vi "ScanPi.vi"() -> ()   [LabVIEW 2019]
uses:
  <vilib>/Platform/TimedLoop/XDataNode/timing_clust.ctl
  <vilib>/Platform/TimedLoop/XDataNode/nitl_modes.ctl
  <vilib>/Platform/TimedLoop/XDataNode/wakeup.ctl
  <vilib>/Analysis/6fits.llb/Curve Fitting Criteria.ctl
  <vilib>/DAQmx/write.llb/DAQmx Write (Analog Wfm 1Chan NSamp).vi
  <vilib>/DAQmx/read.llb/DAQmx Read (Analog Wfm 1Chan NSamp).vi
  <vilib>/Analysis/baseanly.llb/Mean (DBL).vi
  <vilib>/DAQmx/create/channels.llb/DAQmx Create Channel (AO-Voltage-Basic).vi
  <vilib>/DAQmx/configure/timing.llb/DAQmx Timing (Sample Clock).vi
  <vilib>/DAQmx/miscellaneous.llb/DAQmx Fill In Error Info.vi
  <vilib>/DAQmx/create/channels.llb/DAQmx Create Channel (AI-Voltage-Basic).vi
  <vilib>/measure/mascope.llb/Amplitude and Levels 1 chan.vi
  <vilib>/Utility/file.llb/Write Delimited Spreadsheet (DBL).vi
  <vilib>/gmath/NumericalOptimization/Nonlinear Curve Fit LM formula string.vi
  <vilib>/platform/TimedLoop/XDataNode/XDataNode.xnode
  <vilib>/Analysis/NI_AALBase.lvlib
  <vilib>/Platform/TimedLoop/XDataNode/XDNodeRunTimeDep.lvlib
  <vilib>/gmath/NI_Gmath.lvlib
  <vilib>/measure/NI_MABase.lvlib
  <vilib>/measure/NI_MAPro.lvlib
  <vilib>/Analysis/NI_AALPro.lvlib
panel:
  in  "VoltGuess":dbl format="%#_13g"
  in  "file path (dialog if empty)":path=path "C:/Users/Weak/Desktop/May_2018/newAlignment/gpHA_-1185_-1132_31deg.csv"
  in  "stop 2":bool
  in  "Phase":dbl=31.0
  out "In Range?":bool=TRUE
  out "element":dbl=0.7624557364514131
  in  "Ki":dbl=0.15
  in  "Kp":dbl=0.04
  out "m":dbl=-3.5466103770531032
  out "offset":dbl=-1.2655842803924016
  out "Waveform Chart":dynamicdata(graph)=[{"t0"=timestamp(3609575742.2676673 s since 1904-01-01), "dt"=1.0, "Y"=[-6.117337894946104]}, {"t0"=timestamp(3609575742.255667 s since 1904-01-01), "dt"=1.0, "Y"=[-6.086605623645964]}, {"t0"=timestamp(3609575742.2676673 s since 1904-01-01), "dt"=1.0, "Y"=[-1.7123814874696823]}, {"t0"=timestamp(3609575742.2676673 s since 1904-01-01), "dt"=1.0, "Y"=[-0.030732271300140113]}]
  in  "stop":bool
  out "Scanning":waveform(dbl)[](graph)=[{"t0"=timestamp(0 s since 1904-01-01), "dt"=0.000333325, "Y"=array[3000 elements]}, {"t0"=timestamp(0 s since 1904-01-01), "dt"=0.0003333333333333333, "Y"=array[3000 elements]}, {"t0"=timestamp(0 s since 1904-01-01), "dt"=0.000333325, "Y"=array[3000 elements], "attributes"=variant("NI_ChannelName"=variant(string "Filtered (Filtered)"), "NI_OriginalChannelName"=variant(string "Filtered"))}]
  in  "stop Lock":bool
  out "Locking":cluster{"Y":dbl[], "best nonlinear fit":dbl[]}[](graph)=[{"Y"=[-1.2487077639208923], "best nonlinear fit"=[-6.086605623645964]}, {"Y"=array[214 elements], "best nonlinear fit"=array[214 elements]}, {"Y"=array[214 elements], "best nonlinear fit"=array[214 elements]}]
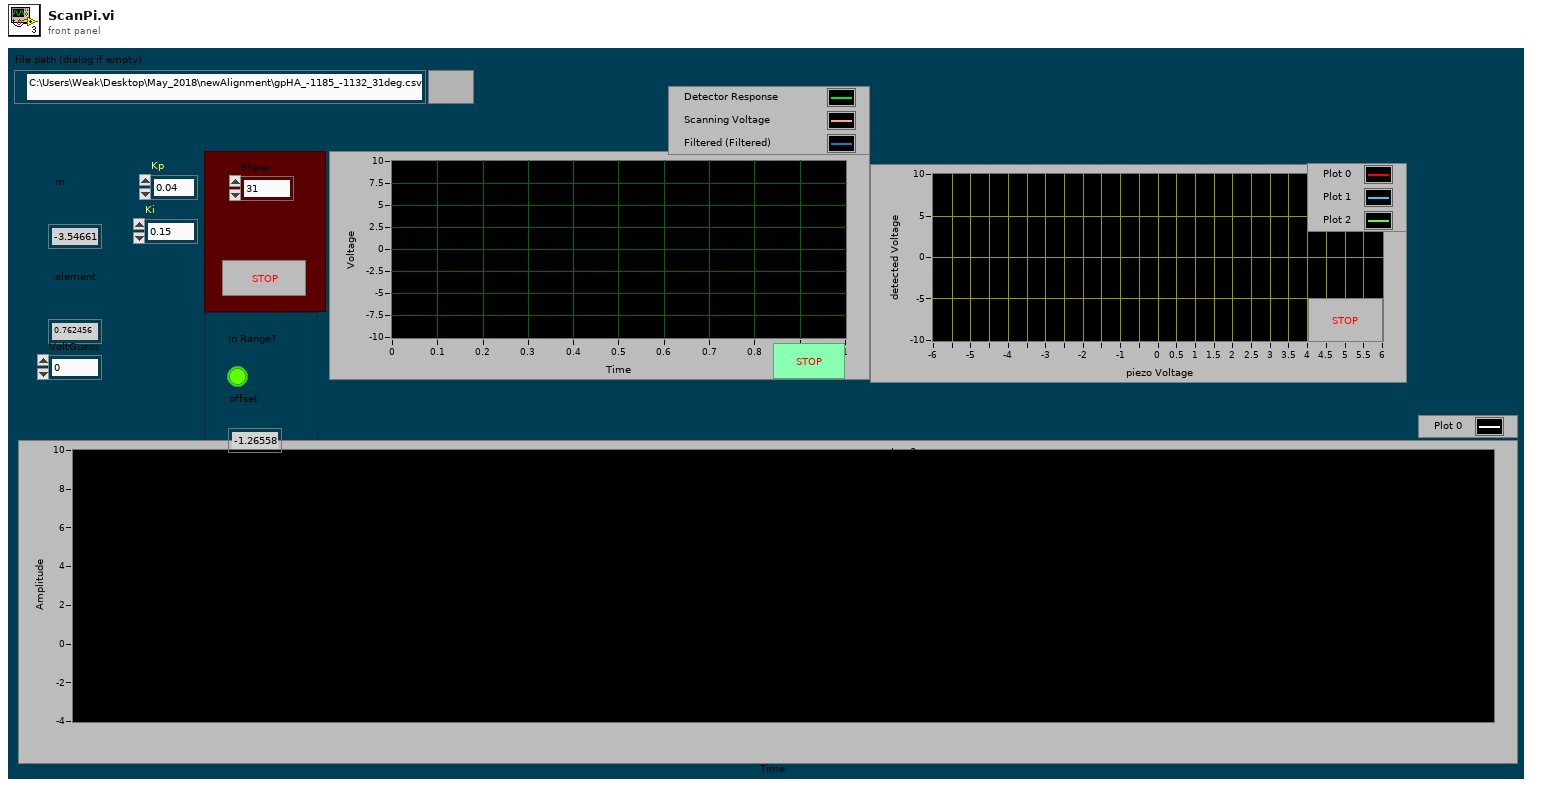
[diagram p1: front panel]
types:
  T1 = enum16{"Sine Wave", "Triangle Wave", "Square Wave", "Sawtooth Wave"}
  T2 = typedef "XDNodeRunTimeDep.lvlib/timing_clust.ctl" = cluster{"Expected End [f-1]":u64, "Actual End [f-1]":u64, "Finished Late? [f-1]":bool, "Expected End [i-1]":u64, "Actual End [i-1]":u64, "Finished Late? [i-1]":bool, "Expected Start [i]":u64, "Actual Start [i]":u64, "Expected Start [f]":u64, "Actual Start [f]":u64, "Source Name":string, "Structure Name":string, "Period":i64, "Deadline":i64, "Offset":i64, "Start":i64, "Priority":i32, "Timeout":i32, "Mode":T3, "Wakeup Reason":T4, "Error":errorcluster, "Source Type":string, "Secondary Source Type":string, "Global End Time":u64, "Global Start Time":u64, "Frame Duration":u64, "Iteration Duration":u64, "Assigned CPU":i32, "I/O Scan Engine Mode":u32}
  T3 = typedef "XDNodeRunTimeDep.lvlib/nitl_modes.ctl" = enum32{"No Change", "Process missed periods, maintain original phase", "Discard missed periods, maintain original phase", "Process missed periods, ignore original phase", "Discard missed periods, ignore original phase"}
  T4 = typedef "XDNodeRunTimeDep.lvlib/wakeup.ctl" = enum32{"Normal", "Aborted", "Asynchronous wakeup", "Timing source error", "Timed loop error", "Timeout"}
  T5 = cluster{"slope min":dbl, "slope max":dbl, "intercept min":dbl, "intercept max":dbl}
  T6 = cluster{"model":string, "Parameters":string[], "x":string}
  T7 = typedef "NI_AALPro.lvlib/Curve Fitting Criteria.ctl" = u16
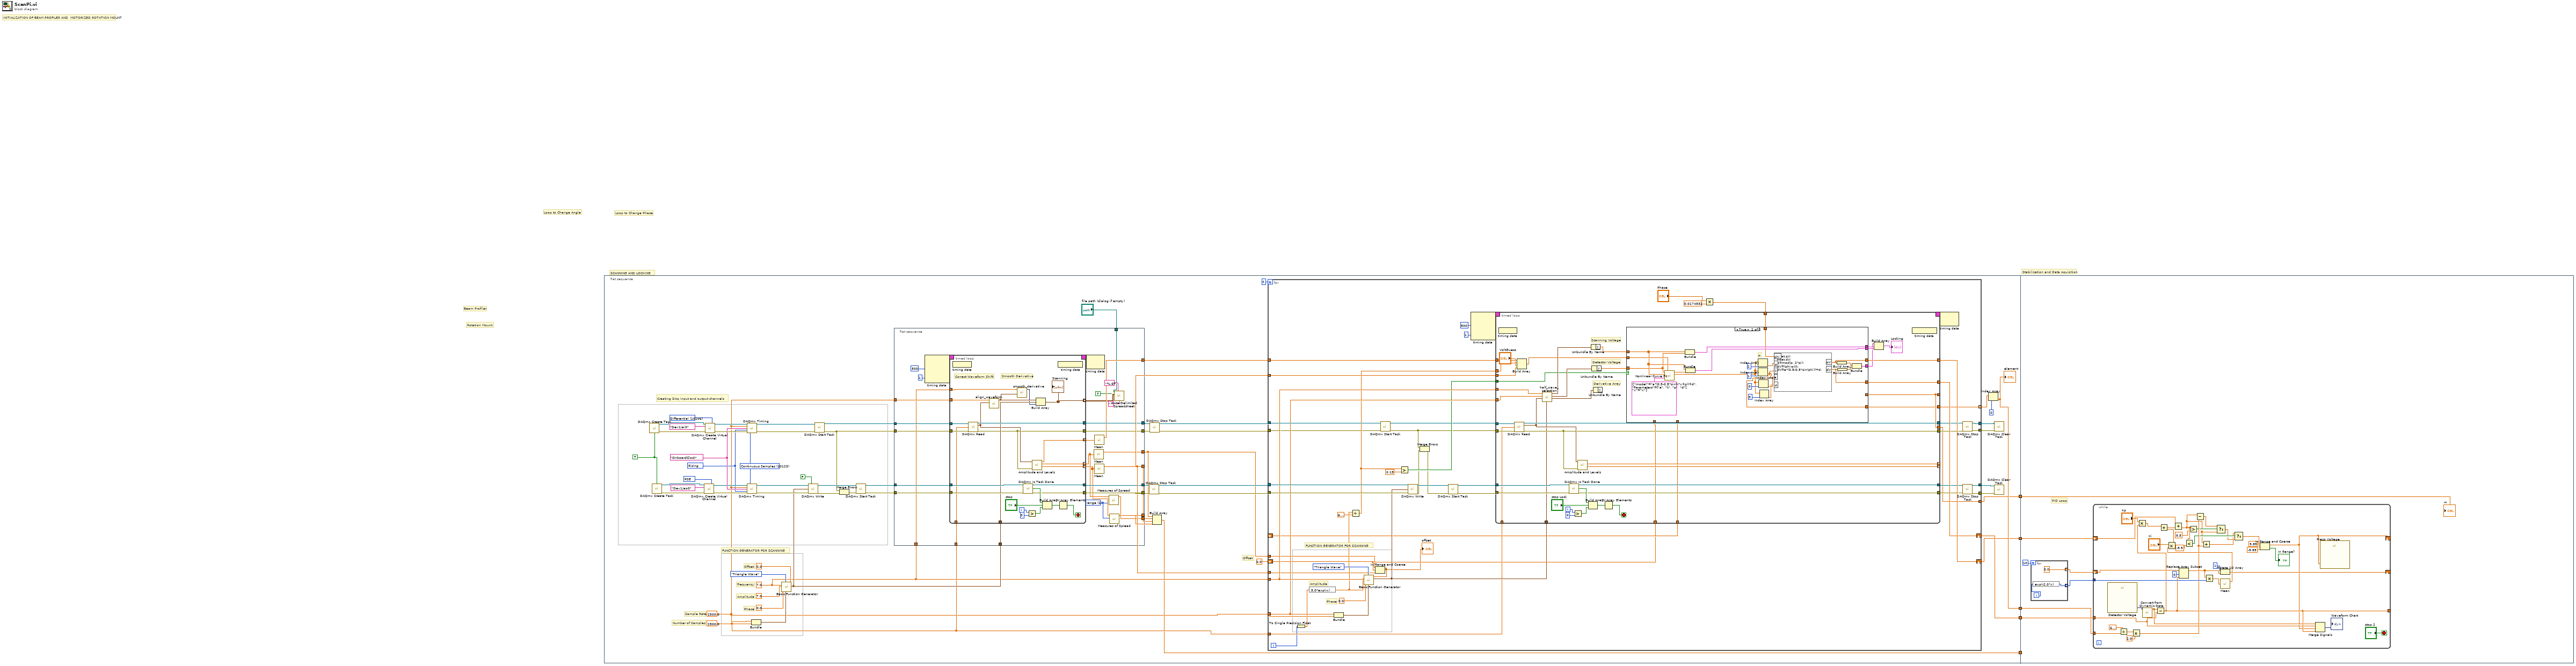
[diagram p0: block diagram]
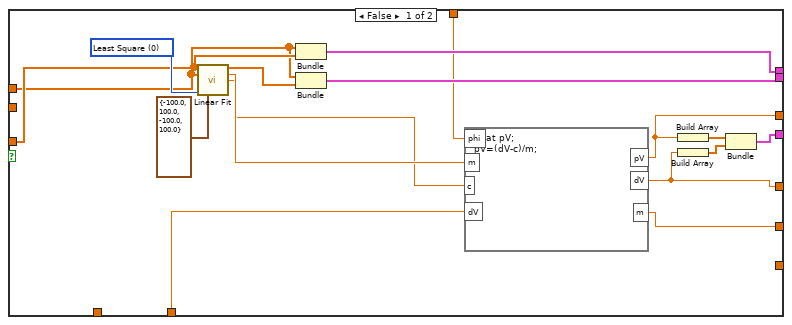
[diagram p2: hidden frame]
diagram:
  # "Stabilization and Data Aquisition"
  # "SCANNING AND LOCKING"
  # "Beam Profiler"
  # "Rotation Mount"
  # "Loop to Change Angle"
  # "Loop to Change Phase"
  # "INITIALIZATION OF BEAM PROFILER AND  MOTORIZED ROTATION MOUNT"
  n1 = flat-sequence {
    tunnel: [w17] -> w5
    tunnel: [w14] -> w4
    tunnel: [w13] -> w3
    tunnel: [w10] -> w2
    tunnel: [w9] -> w1
    tunnel: w5 -> [w280]
    tunnel: w4 -> [_]
    tunnel: w3 -> [w279]
    tunnel: w2 -> [w275]
    tunnel: w1 -> [w274]
    frame #0 {
      w33 = TRUE ("auto cleanup")
      w19 = 2500.0
      w20 = 7.0 ("frequency")
      w59 = 10123 items=["Finite Samples"=10178, "Continuous Samples"=10123, "Hardware Timed Single Point"=12522] ("sample mode")
      w18 = 2500.0
      w60 = 10280 items=["Rising"=10280, "Falling"=10171] ("active edge")
      w65 = tag "OnboardClock" ("source")
      w66 = 10083 items=["Default"=-1, "RSE"=10083, "Differential"=10106, "Pseudodifferential"=12529] ("output terminal configuration")
      w68 = 10106 items=["Default"=-1, "RSE"=10083, "NRSE"=10078, "Differential"=10106, "Pseudodifferential"=12529] ("input terminal configuration")
      # "Number of Samples"
      # "FUNCTION GENERATOR FOR SCANNING"
      # "Phase"
      # "Amplitude"
      # "Frequency"
      # "Offset"
      # "Sample Rate"
      # "Creating DAq input and output channels"
      # "Offset"
      n2 = call <vilib>:"DAQmx Create Task.vi"("auto cleanup"=w33) -> ("task out"=w36:refnum<k21>, "error out"=w35:errorcluster)  [unwired: 13 in]
      n3 = call <vilib>:"DAQmx Create Task.vi"("auto cleanup"=w33) -> ("task out"=w34:refnum<k21>, "error out"=w32:errorcluster)  [unwired: 13 in]
      n4 = call-poly <vilib>:"DAQmx Create Virtual Channel.vi"("task in"=w34, "output terminal configuration"=w66, "physical channels"=tag "Dev1/ao0", "error in"=w32) -> ("task out"=w62:refnum<k21>, "error out"=w61:errorcluster)  [unwired: 10 in]
      n5 = call-poly <vilib>:"DAQmx Create Virtual Channel.vi"("task in"=w36, "input terminal configuration"=w68, "physical channels"=tag "Dev1/ai0", "error in"=w35) -> ("task out"=w64:refnum<k21>, "error out"=w63:errorcluster)  [unwired: 10 in]
      n6 = call-poly <vilib>:"DAQmx Timing.vi"("task/channels in"=w64, "sample mode"=w59, "rate"=w18, "source"=w65, "active edge"=w60, "error in"=w63) -> ("task out"=w50:refnum<k21>, "error out"=w49:errorcluster)  [unwired: 8 in]
      n7 = call-poly <vilib>:"DAQmx Timing.vi"("task/channels in"=w62, "sample mode"=w59, "rate"=w18, "source"=w65, "active edge"=w60, "error in"=w61) -> ("task out"=w58:refnum<k21>, "error out"=w57:errorcluster)  [unwired: 8 in]
      n8 = Bundle(w18, w19) -> (w52:cluster{dbl, dbl})  [unwired: 1 in]
      n9 = call <vilib>:"Basic Function Generator.vi"("offset"=0.0, "sampling info"=w52, "signal type"=T1."Triangle Wave", "phase"=0.0, "amplitude"=7.0, "frequency"=w20) -> ("signal out"=w47:waveform(dbl))  [unwired: 3 in, 2 out]
      n10 = call-poly <vilib>:"DAQmx Write.vi"("task/channels in"=w58, "auto start"=FALSE, "data"=w47, "error in"=w57) -> ("task out"=w51:refnum<k21>, "error out"=w42:errorcluster)  [unwired: 9 in, 1 out]
      n11 = call <vilib>:"DAQmx Start Task.vi"("task/channels in"=w50, "error in"=w49) -> ("task out"=w48:refnum<k21>, "error out"=w43:errorcluster)  [unwired: 12 in]
      n12 = Merge Errors(w43, w42) -> (w44:errorcluster)
      n13 = call <vilib>:"DAQmx Start Task.vi"("task/channels in"=w51, "error in"=w44) -> ("task out"=w45:refnum<k21>, "error out"=w46:errorcluster)  [unwired: 12 in]
      n14 = flat-sequence {
        tunnel: w48 -> [w97]
        tunnel: w43 -> [w96]
        tunnel: w47 -> [w95]
        tunnel: w46 -> [w94]
        tunnel: w45 -> [w93]
        tunnel: w18 -> [w91]
        tunnel: w19 -> [w90]
        tunnel: w20 -> [w89]
        tunnel: [w88] -> w38
        tunnel: [w87] -> w40
        tunnel: [w86] -> w39
        tunnel: [w85] -> w37
        tunnel: [w83] -> w23
        tunnel: [w82] -> w8
        tunnel: [w81] -> w7
        tunnel: [w76] -> w16
        tunnel: [w75] -> w15
        tunnel: "file path (dialog if empty)" -> [w71]
        frame #0 {
          w77 = 1 items=["standard deviation", "range", "mean absolute deviation", "interquartile range"] ("type")
          n15 = node-c288(i64 500 ("Period"), 1 ("Processor")) -> (w99:T2)  [unwired: 2 in]
          n16 = timed-loop {
            timing: w99 -> [_]
            timing-out: [_] -> w98
            tunnel: w97 -> [w125]
            tunnel: w96 -> [w124]
            tunnel: w95 -> [w111]
            tunnel: w94 -> [w113]
            tunnel: w93 -> [w123]
            tunnel: [w115] -> w88
            tunnel: [w105] -> w85
            tunnel: [w114] -> w87
            tunnel: [w112] -> w86
            tunnel: w91 -> [w110]
            tunnel: w90 -> [w109]
            tunnel: w89 -> [w107]
            tunnel: [w104] -> w79 mode=indexing
            tunnel: [w103] -> w78 mode=indexing
            tunnel: [w102] -> w84 mode=indexing
            tunnel: [w100] -> w74 mode=indexing
            i -> [w120]
            stop <- w116 stop-if-true
            # "Smooth Derivative"
            # "Correct Waveform Shift"
            n17 = node-c288() -> ()  [unwired: 1 in]
            n18 = call-poly <vilib>:"DAQmx Read.vi"("task/channels in"=w125, "number of samples per channel"=w109, "error in"=w124) -> ("task out"=w115:refnum<k21>, "data"=w106:waveform(dbl), "error out"=w105:errorcluster)  [unwired: 10 in]
            n19 = call "align_waveform.vi"("Input Waveform"=w106, "Sample Rate to be Wired"=w110) -> ("Output Waveform"=w108:waveform(dbl))  [unwired: 9 in]
            n20 = call "smooth_derivative.vi"("Output Waveform"=w108, "frequency"=w107) -> ("Filtered Signal"=w101:dynamicdata)  [unwired: 9 in]
            n21 = call <vilib>:"DAQmx Is Task Done.vi"("task/channels in"=w123, "error in"=w113) -> ("task out"=w114:refnum<k21>, "task done?"=w121:bool, "error out"=w112:errorcluster)  [unwired: 11 in]
            n22 = Greater?(x=w120, y=3) -> (0:w117:bool)
            n23 = call-poly <vilib>:"Amplitude and Levels.vi"("error in (no error)"=w105, "signal in"=w106) -> ("low state level"=w103:dbl, "high state level"=w104:dbl, "amplitude"=w102:dbl)  [unwired: 6 in, 1 out]
            n24 = Build Array(w108, w111, w101) -> (w100:waveform(dbl)[])
            "Scanning" <- w100
            n25 = Build Array(w121, "stop", w117) -> (w122:bool[])
            n26 = node-c288() -> ()  [unwired: 1 out]
            n27 = Or Array Elements(Boolean array=w122) -> (logical OR=w116:bool)
          }
          n28 = node-c288(w98) -> ()  [unwired: 1 out]
          n29 = call-poly <vilib>:"Mean.vi"("X"=w79) -> ("mean"=w82:dbl)  [unwired: 1 out]
          n30 = call-poly <vilib>:"Mean.vi"("X"=w84) -> ("mean"=w83:dbl)  [unwired: 1 out]
          n31 = call-poly <vilib>:"Mean.vi"("X"=w78) -> ("mean"=w81:dbl)  [unwired: 1 out]
          n32 = call <vilib>:"Measures of Spread.vi"("type"=w77, "x array"=w79) -> ("spread value"=w76:dbl)  [unwired: 8 in, 1 out]
          n33 = call <vilib>:"Measures of Spread.vi"("type"=w77, "x array"=w78) -> ("spread value"=w75:dbl)  [unwired: 8 in, 1 out]
          n34 = call-poly <vilib>:"Write Delimited Spreadsheet.vi"("file path (dialog if empty)"=w71, "format (%.3f)"="%.6f", "2D data"=w74, "transpose? (no:F)"=TRUE, "delimiter (\\t)"="," ("delimiter (\\t)")) -> ()  [unwired: 9 in, 2 out]
        }
      }
      n35 = call <vilib>:"DAQmx Stop Task.vi"("task/channels in"=w40, "error in"=w39) -> ("task out"=w22:refnum<k21>, "error out"=w21:errorcluster)  [unwired: 12 in]
      n36 = call <vilib>:"DAQmx Stop Task.vi"("task/channels in"=w38, "error in"=w37) -> ("task out"=w25:refnum<k21>, "error out"=w24:errorcluster)  [unwired: 12 in]
      n37 = Build Array(w8, w16, w7, w15) -> (w14:dbl[])
      n38 = for {
        N: 4 -> [_]
        tunnel: w19 -> [w175]
        tunnel: w20 -> [w173]
        tunnel: w18 -> [w172]
        tunnel: w23 -> [w171]
        tunnel: w7 -> [w170]
        tunnel: w25 -> [w174]
        tunnel: w24 -> [w150]
        tunnel: w22 -> [w181]
        tunnel: w21 -> [w180]
        shift-right: [w165] -> w9
        shift-left: 0.0 ("offset") -> [w139]
        shift-right: [w159] -> w17
        shift-left: _ -> [w158]
        tunnel: [w147] -> w27
        tunnel: [w146] -> w26
        tunnel: [w143] -> w29
        tunnel: [w142] -> w28
        tunnel: [w141] -> w12 mode=indexing
        tunnel: [w140] -> w10
        tunnel: w8 -> [w138]
        tunnel: w7 -> [w137]
        i -> [w167]
        # "FUNCTION GENERATOR FOR SCANNING"
        # "Phase"
        # "Amplitude"
        n39 = To Single Precision Float(number=w167) -> (single precision float=w166:sgl)
        n40 = expression code="5.0*exp(-x)"(w166) -> (w168:sgl)
        n41 = Bundle(w172, w175) -> (w177:cluster{dbl, dbl})  [unwired: 1 in]
        n42 = Divide(x=w168, y=6.283185307179586) -> (x/y=w162:dbl)
        n43 = In Range and Coerce(upper limit=w138, x=w139, lower limit=w137) -> (coerced(x)=w136:dbl)  [unwired: 1 out]
        "offset" <- w136
        n44 = call <vilib>:"Basic Function Generator.vi"("offset"=w136, "sampling info"=w177, "signal type"=T1."Triangle Wave", "phase"=0.0, "amplitude"=w168, "frequency"=w173) -> ("signal out"=w176:waveform(dbl))  [unwired: 3 in, 2 out]
        n45 = call <vilib>:"DAQmx Start Task.vi"("task/channels in"=w174, "error in"=w150) -> ("task out"=w152:refnum<k21>, "error out"=w151:errorcluster)  [unwired: 12 in]
        n46 = Greater?(x=w162, y=0.15) -> (0:w160:bool)
        n47 = call-poly <vilib>:"DAQmx Write.vi"("task/channels in"=w181, "data"=w176, "error in"=w180) -> ("task out"=w155:refnum<k21>, "error out"=w154:errorcluster)  [unwired: 10 in, 1 out]
        n48 = Merge Errors(w151, w154) -> (w153:errorcluster)
        n49 = call <vilib>:"DAQmx Start Task.vi"("task/channels in"=w155, "error in"=w153) -> ("task out"=w157:refnum<k21>, "error out"=w156:errorcluster)  [unwired: 12 in]
        n50 = node-c288(i64 500 ("Period"), 1 ("Processor")) -> (w183:T2)  [unwired: 2 in]
        n51 = Multiply(x="Phase", y=0.0174532) -> (x*y=w134:dbl)
        n52 = timed-loop {
          timing: w183 -> [_]
          timing-out: [_] -> w182
          tunnel: w152 -> [w227]
          tunnel: w151 -> [w226]
          tunnel: w176 -> [w206]
          tunnel: w156 -> [w215]
          tunnel: w157 -> [w225]
          tunnel: [w217] -> w145
          tunnel: [w211] -> w144
          tunnel: [w216] -> w149
          tunnel: [w214] -> w148
          tunnel: w172 -> [w208]
          tunnel: w175 -> [w213]
          tunnel: w173 -> [w207]
          tunnel: [w210] -> _ mode=indexing
          tunnel: [w209] -> _ mode=indexing
          tunnel: w171 -> [w202]
          tunnel: w170 -> [w193]
          tunnel: w162 -> [w201]
          tunnel: w134 -> [w192]
          tunnel: [w190] -> w165
          tunnel: w160 -> [w189]
          tunnel: w139 -> [w188]
          tunnel: [w187] -> w159
          tunnel: w158 -> [w186]
          tunnel: [w185] -> w141
          tunnel: [w184] -> _
          tunnel: [w184] -> w140
          i -> [w222]
          stop <- w218 stop-if-true
          # "Derivative Array"
          # "Detector Voltage"
          # "Scanning Voltage"
          n53 = node-c288() -> ()  [unwired: 1 in]
          n54 = call-poly <vilib>:"DAQmx Read.vi"("task/channels in"=w227, "number of samples per channel"=w213, "error in"=w226) -> ("task out"=w217:refnum<k21>, "data"=w212:waveform(dbl), "error out"=w211:errorcluster)  [unwired: 10 in]
          n55 = Build Array(w202, w201, "VoltGuess", w193) -> (w200:dbl[])
          n56 = call "half_wave_selection.vi"("signal in"=w206, "data"=w212, "Numeric"=w208, "frequency"=w207) -> ("waveform out"=w203:waveform(dbl), "waveform out 2"=w204:waveform(dbl), "waveform out 3"=w205:waveform(dbl))  [unwired: 5 in]
          n57 = call <vilib>:"DAQmx Is Task Done.vi"("task/channels in"=w225, "error in"=w215) -> ("task out"=w216:refnum<k21>, "task done?"=w223:bool, "error out"=w214:errorcluster)  [unwired: 11 in]
          n58 = Greater?(x=w222, y=0) -> (0:w219:bool)
          n59 = call-poly <vilib>:"Amplitude and Levels.vi"("error in (no error)"=w211, "signal in"=w212) -> ("low state level"=w209:dbl, "high state level"=w210:dbl)  [unwired: 6 in, 2 out]
          n60 = Build Array(w223, "stop Lock", w219) -> (w224:bool[])
          n61 = Unbundle By Name(w205) -> ("Y"=w199:dbl[])
          n62 = Unbundle By Name(w204) -> ("Y"=w198:dbl[])
          n63 = Unbundle By Name(w203) -> ()  [unwired: 1 out]
          n64 = Or Array Elements(Boolean array=w224) -> (logical OR=w218:bool)
          n65 = case shown="True" w189 {
            tunnel: w200 -> [_ w265]
            tunnel: w199 -> [w240 w263]
            tunnel: w198 -> [w242 w262]
            tunnel: [w241 w261] -> w197
            tunnel: [w238 w260] -> w196
            tunnel: w192 -> [w236 w259]
            tunnel: [w232 w249] -> w191
            tunnel: [w229 w248] -> w190
            tunnel: w188 -> [_ _]
            tunnel: [w230 w247] -> w187
            tunnel: w186 -> [w233 _]
            tunnel: [_ w245] -> w185
            tunnel: [w228 _] -> w184
            frame False {
              w244 = T7 0 items=["Least Square", "Least Absolute Residual", "Bisquare"] ("method")
              n66 = call <vilib>:"Linear Fit.vi"("Y"=w242, "X"=w240, "method"=w244, "parameter bounds"=T5 {"slope min"=-100.0, "slope max"=100.0, "intercept min"=-100.0, "intercept max"=100.0}) -> ("Best Linear Fit"=w239:dbl[], "slope"=w235:dbl, "intercept"=w234:dbl)  [unwired: 7 in, 2 out]
              n67 = Bundle("Y"=w240, "Y"=w242) -> (w241:cluster{"Y":dbl[], "Y":dbl[]})  [unwired: 1 in]
              n68 = Bundle("Y"=w240, "Best Linear Fit"=w239) -> (w238:cluster{"Y":dbl[], "Best Linear Fit":dbl[]})  [unwired: 1 in]
              n69 = formula code="float pV;\npV=(dV-c)/m;"("phi"=w236, "m"=w235, "c"=w234, "dV"=w233) -> ("pV"=w229:dbl, "dV"=w230:dbl, "m"=w228:dbl)
              n70 = Build Array(w229) -> (w231:dbl[])
              n71 = Build Array(w230) -> (w237:dbl[])
              n72 = Bundle(w231, w237) -> (w232:cluster{dbl[], dbl[]})  [unwired: 1 in]
            }
            frame True {
              # "p"
              n73 = call-poly <vilib>:"Nonlinear Curve Fit.vi"("Y"=w262, "initial parameters"=w265, "X"=w263, "model description"=T6 {"model"="a*(0.5-0.5*sin(k*x+p))+d", "Parameters"=["a", "k", "p", "d"], "x"="x"}) -> ("best nonlinear fit"=w264:dbl[], "best fit parameters"=w253:dbl[])  [unwired: 7 in, 3 out]
              n74 = Bundle("Y"=w263, "Y"=w262) -> (w261:cluster{"Y":dbl[], "Y":dbl[]})  [unwired: 1 in]
              n75 = Bundle("Y"=w263, "best nonlinear fit"=w264) -> (w260:cluster{"Y":dbl[], "best nonlinear fit":dbl[]})  [unwired: 1 in]
              n76 = Index Array(array=w253, index=2) -> (element=w256:dbl)
              n77 = Index Array(array=w253, index=1) -> (element=w245:dbl)
              n78 = Index Array(array=w253, index=0) -> (element=w255:dbl)
              n79 = Index Array(array=w253, index=3) -> (element=w246:dbl)
              n80 = formula code="float pV;\nfloat dV;\np=mod(p, 2*pi);\npV=(phi-p)/k;\ndV=a*(0.5-0.5*sin(phi))+d;"("phi"=w259, "p"=w256, "k"=w245, "a"=w255, "d"=w246) -> ("pV"=w248:dbl, "dV"=w247:dbl)
              n81 = Build Array(w248) -> (w251:dbl[])
              n82 = Build Array(w247) -> (w250:dbl[])
              n83 = Bundle(w251, w250) -> (w249:cluster{dbl[], dbl[]})  [unwired: 1 in]
            }
          }
          n84 = Build Array(w191, w197, w196) -> (→"Locking":cluster{"Y":dbl[], "best nonlinear fit":dbl[]}[])
          n85 = node-c288() -> ()  [unwired: 1 out]
        }
        n86 = node-c288(w182) -> ()  [unwired: 1 out]
        n87 = call <vilib>:"DAQmx Stop Task.vi"("task/channels in"=w145, "error in"=w144) -> ("task out"=w143:refnum<k21>, "error out"=w142:errorcluster)  [unwired: 12 in]
        n88 = call <vilib>:"DAQmx Stop Task.vi"("task/channels in"=w149, "error in"=w148) -> ("task out"=w147:refnum<k21>, "error out"=w146:errorcluster)  [unwired: 12 in]
      }
      n89 = Index Array(array=w12, index=0) -> (element=w13:dbl)
      "element" <- w13
      n90 = call <vilib>:"DAQmx Clear Task.vi"("task in"=w29, "error in"=w28) -> ()  [unwired: 13 in, 1 out]
      n91 = call <vilib>:"DAQmx Clear Task.vi"("task in"=w27, "error in"=w26) -> ()  [unwired: 13 in, 1 out]
    }
    frame #1 {
      # "PID Loop"
      n92 = for {
        N: 10 -> [_]
        tunnel: [w320] -> w276 mode=indexing
        tunnel: [0.0] -> w277 mode=indexing
        i -> [w321]
        n93 = expression code="exp(-2.0*x)"(w321) -> (w320:i32)
      }
      n94 = while {
        tunnel: w280 -> [w281]
        tunnel: w279 -> [w282]
        shift-right: [w311] -> _
        shift-left: w277 -> [w314]
        tunnel: w276 -> [w309]
        tunnel: [w293] -> _
        shift-right: [w287] -> _
        shift-left: w274 -> [w290]
        stop <- "stop 2" stop-if-true
        n95 = call "Detector Voltage"() -> ("data"=w307:dynamicdata)  [unwired: 17 in, 2 out]
        n96 = Divide(x=6.283185307179586, y=w282) -> (x/y=w316:dbl)
        n97 = Multiply(x=w316, y=2.0) -> (x*y=w301:dbl)
        n98 = call "Convert from Dynamic Data"("Dynamic Data Type"=w307) -> ("Scalar"=w292:dbl)  [unwired: 3 in]
        n99 = Subtract(x=w292, y=w281) -> (x-y=w293:dbl)
        n100 = Multiply(x="Kp", y=w293) -> (x*y=w303:dbl)
        n101 = Replace Array Subset(array=w314, new element=w293, index=0) -> (w310:dbl[])
        n102 = Multiply(x=w310, y=w309) -> (x*y=w308:dbl[])
        n103 = call-poly <vilib>:"Mean.vi"("X"=w308) -> ("mean"=w304:dbl)  [unwired: 1 out]
        n104 = Multiply(x="Ki", y=w304) -> (x*y=w302:dbl)
        n105 = Add(x=w303, y=w302) -> (x+y=w297:dbl)
        n106 = Add(x=w290, y=w297) -> (x+y=w291:dbl)
        n107 = Less?(x=w291, y=-9.5) -> (x < y?=w296:bool)
        n108 = Greater?(x=w291, y=9.5) -> (0:w300:bool)
        n109 = Subtract(x=w291, y=w301) -> (x-y=w299:dbl)
        n110 = Add(x=w291, y=w301) -> (x+y=w295:dbl)
        n111 = Select(t=w299, s=w300, f=w291) -> (s? t:f=w294:dbl)
        n112 = Rotate 1D Array(1:w310, 2:1 ("n")) -> (0:w311:dbl[])
        n113 = Select(t=w295, s=w296, f=w294) -> (s? t:f=w288:dbl)
        n114 = In Range and Coerce(upper limit=9.85, x=w288, lower limit=-9.85) -> (coerced(x)=w287:dbl, In Range?=→"In Range?":bool)
        n115 = Merge Signals(w292, w281, w287, w293) -> (→"Waveform Chart":dynamicdata)
        n116 = call "Piezo Voltage"("data"=w287) -> ()  [unwired: 17 in, 2 out]
      }
      "m" <- w275
    }
  }
